vi "Remove.vi"(8 "error in (no error)":errorcluster, 10 "key":string, 11 "Object Dictionary in":refnum<class "objdict.lvclass">) -> (0 "error out":errorcluster, 1 "Object":refnum<class>, 2 "found":bool, 3 "Object Dictionary out":refnum<class "objdict.lvclass">)   [LabVIEW 2015, in "objdict.lvclass"]
doc: "If an object is assigned to the specified key in the dictionary, this VI removes it from the dictionary and destroys its Data Value Reference. The removed object is returned by this VI."
uses:
  objdict.lvclass
  objdict.lvclass/objdict.ctl
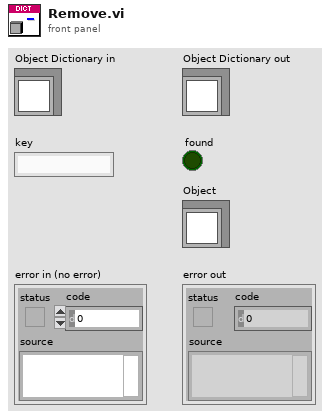
[diagram p1: front panel]
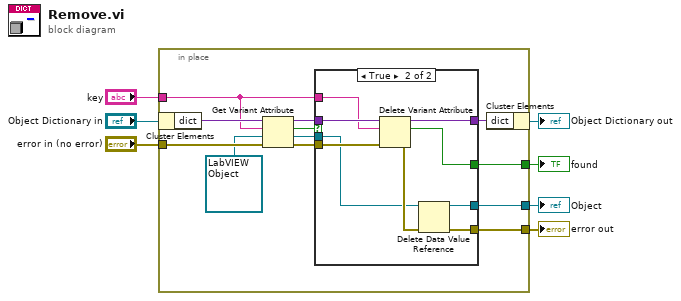
[diagram p0: block diagram]
diagram:
  n1 = in-place {
    in-place-border: [w12] -> w5
    in-place-border: "error in (no error)" -> [w19]
    in-place-border: "key" -> [w14]
    in-place-border: [w10] -> w2
    in-place-border: [w8] -> w1
    n2 = in-place-cluster #1("Object Dictionary in") -> ("dict"=w16:variant)
    n3 = Get Variant Attribute(Variant=w16, name=w14, default value (empty Variant)=refnum<data-value> refnum ("data value reference"), error in=w19) -> (duplicate Variant=w15:variant, found=w9:bool, value=w11:refnum<data-value>, error out=w17:errorcluster)
    n4 = case shown="True" w9 {
      selector: w9 -> [w20 _]
      tunnel: [w21 w30] -> w18
      tunnel: w17 -> [w22 w29]
      tunnel: w15 -> [w21 w28]
      tunnel: w14 -> [_ w27]
      tunnel: [w22 w26] -> w12
      tunnel: w11 -> [_ w25]
      tunnel: [_ w24] -> w10
      tunnel: [w20 w23] -> w8
      frame False {
      }
      frame True {
        n5 = Delete Variant Attribute(4:w29, 6:w27, 7:w28) -> (0:w31:errorcluster, 2:w23:bool, 3:w30:variant)
        n6 = Delete Data Value Reference(data value reference=w25, error in=w31) -> (data value=w24:refnum<class>, error out=w26:errorcluster)
      }
    }
    n7 = in-place-cluster #1("dict"=w18) -> (→"Object Dictionary out":refnum<class "objdict.lvclass">)
  }
  "error out" <- w5
  "Object" <- w2
  "found" <- w1
